vi "Set best focus.vi"(8 "error in (no error)":errorcluster, 9 "focus quality":dbl, 10 "best focus":dbl, 11 "Autofocus in":refnum<class "Autofocus.lvclass">) -> (0 "error out":errorcluster, 3 "Autofocus out":refnum<class "Autofocus.lvclass">)   [LabVIEW 2012, in "Autofocus.lvclass"]
uses:
  Autofocus.lvclass
  Autofocus.lvclass/Autofocus.ctl
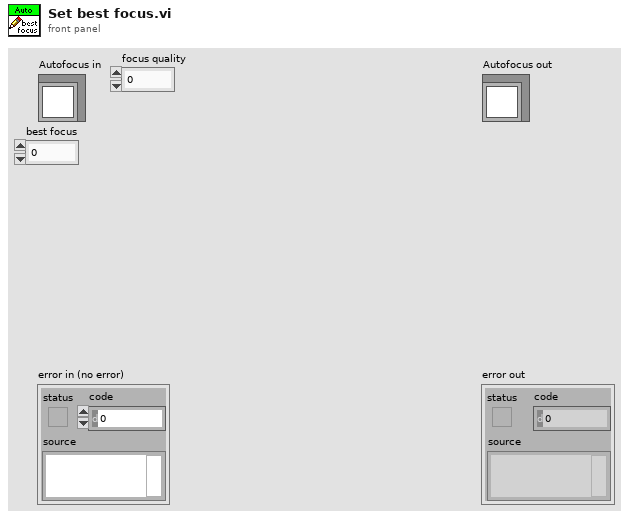
[diagram p1: front panel]
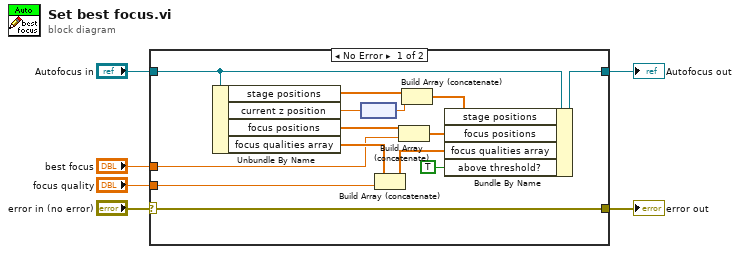
[diagram p0: block diagram]
diagram:
  n1 = case shown="No Error" "error in (no error)" {
    selector: "error in (no error)" -> [w20 w22]
    tunnel: [w20 w22] -> w5
    tunnel: [w19 w21] -> w3
    tunnel: "Autofocus in" -> [w18 w21]
    tunnel: "focus quality" -> [w9 _]
    tunnel: "best focus" -> [w8 _]
    frame No Error {
      n2 = Unbundle By Name(w18) -> ("stage positions"=w17:dbl[], "current z position"=w16:dbl[unit], "focus positions"=w12:dbl[], "focus qualities array"=w11:dbl[])
      n3 = node(w16) -> (w15:dbl)
      n4 = Build Array (concatenate)(w11, w9) -> (w10:dbl[])
      n5 = Build Array (concatenate)(w12, w8) -> (w13:dbl[])
      n6 = Build Array (concatenate)(w17, w15) -> (w14:dbl[])
      n7 = Bundle By Name(cluster=w18, "stage positions"=w14, "focus positions"=w13, "focus qualities array"=w10, "above threshold?"=TRUE ("Runtime cluster.Stack.above threshold?")) -> (w19:refnum<class "Autofocus.lvclass">)
    }
    frame Error {
    }
  }
  "error out" <- w5
  "Autofocus out" <- w3
